vi "init.vi"(8 "error in (no error)":errorcluster, 11 "AmbientTemperatureSensor in":refnum<class "AmbientTemperatureSensor.lvclass">) -> (0 "error out":errorcluster, 3 "AmbientTemperatureSensor out":refnum<class "AmbientTemperatureSensor.lvclass">)   [LabVIEW 2013, in "AmbientTemperatureSensor.lvclass"]
uses:
  AmbientTemperatureSensor.lvclass
  Configuration/AmbientTemperatureSensor.ctl
  <userlib>/Common/SerialProtocols/Configuration/SerialConfig.ctl
  <userlib>/Common/SerialProtocols/Configuration/SerialProtocol.ctl
  <userlib>/Common/SerialProtocols/Configuration/ProtocolParameters.ctl
  <userlib>/Common/SerialProtocols/Configuration/SerialMessageParameters.ctl
  <userlib>/Common/Devices/TemperatureSensor/TemperatureSensor/TemperatureSensor.lvclass/TemperatureSensor.ctl
  ConfigurationThisComponent/ConfigurationThisComponent.lvclass
  <userlib>/Common/SerialProtocols/SerialProtocols.lvlib
  <userlib>/Common/Devices/TemperatureSensor/TemperatureSensor/TemperatureSensor.lvclass
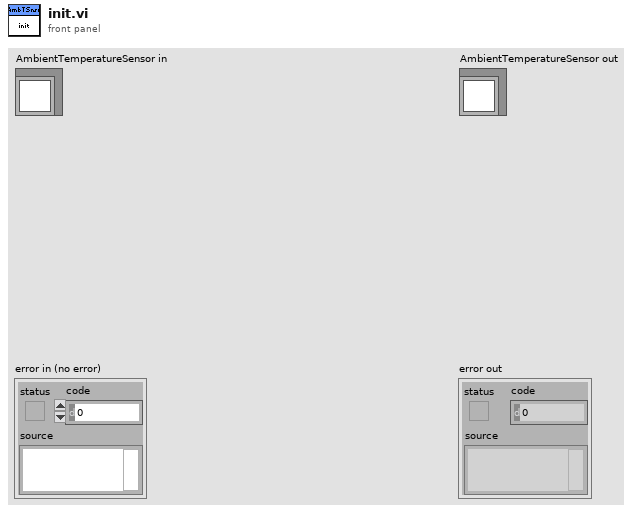
[diagram p1: front panel]
types:
  T1 = typedef "AmbientTemperatureSensor.ctl" = cluster{"Serial":T2}
  T2 = typedef "SerialProtocols.lvlib/SerialConfig.ctl" = cluster{"Serial Protocol":T3, "Protocol Parameters":T4, "Serial Message Parameters":T5}
  T3 = typedef "SerialProtocols.lvlib/SerialProtocol.ctl" = enum16{"RS232", "RS485", "SerialSimulator"}
  T4 = typedef "SerialProtocols.lvlib/ProtocolParameters.ctl" = cluster{"VISA resource name":refnum<visa-resource-name>, "Baud Rate":u32, "Data Bits":u16, "Parity":enum16{"None", "Odd", "Even", "Mark", "Space"}, "Flow Control":u16, "Stop Bits":u16, "Timeout (ms)":u32}
  T5 = typedef "SerialProtocols.lvlib/SerialMessageParameters.ctl" = cluster{"Byte Count":u32, "Enable Termination Character":bool, "Termination Char":u8}
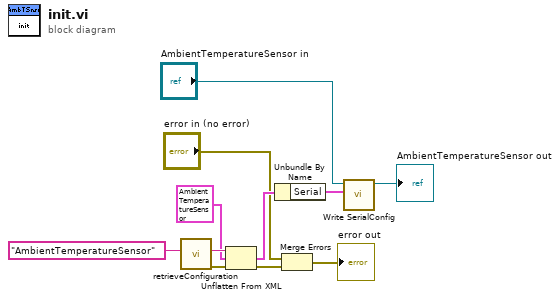
[diagram p0: block diagram]
diagram:
  n1 = call "retrieveConfiguration.vi"("configName"="AmbientTemperatureSensor") -> ("error out"=w8:errorcluster, "xmlConfig"=w9:string)  [unwired: 8 in, 1 out]
  n2 = Unflatten From XML(xml string=w9, type=T1 {"Serial"={"Serial Protocol"=enum."RS232", "Protocol Parameters"={"VISA resource name"="", "Baud Rate"=0, "Data Bits"=0, "Parity"=enum."None", "Flow Control"=0, "Stop Bits"=0, "Timeout (ms)"=0}, "Serial Message Parameters"={"Byte Count"=0, "Enable Termination Character"=FALSE, "Termination Char"=0}}} ("Ambient Temperature Sensor"), error in (no error)=w8) -> (value=w6:T1, error out=w11:errorcluster)
  n3 = Unbundle By Name(w6) -> ("Serial"=w3:T2)
  n4 = Merge Errors("error in (no error)", w11) -> (→"error out":errorcluster)
  n5 = call <userlib>:"Write SerialConfig.vi"("SerialConfig"=w3, "TemperatureSensor in"="AmbientTemperatureSensor in") -> ("TemperatureSensor out"=→"AmbientTemperatureSensor out":refnum<class "AmbientTemperatureSensor.lvclass">)  [unwired: 9 in]
